vi "get_schemas.vi"(8 "error in (no error)":errorcluster, 11 "DB Session ID":i32) -> (0 "error out":errorcluster, 2 "Schemas":string[](array[string]), 3 "DB Session ID out":i32)   [LabVIEW 2017, in "Database.lvlib"]
uses:
  Database.lvlib
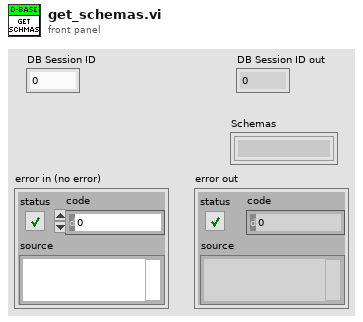
[diagram p1: front panel]
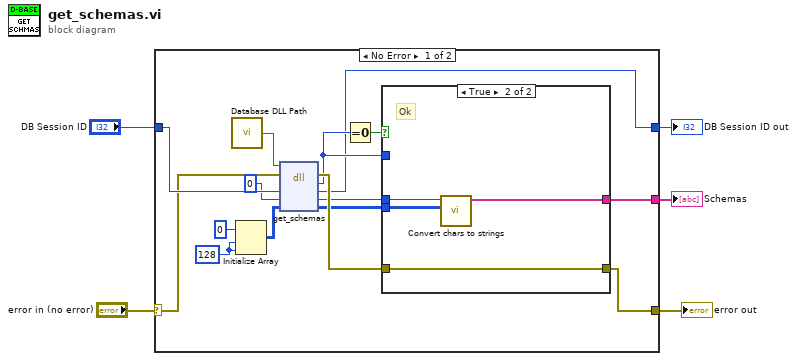
[diagram p0: block diagram]
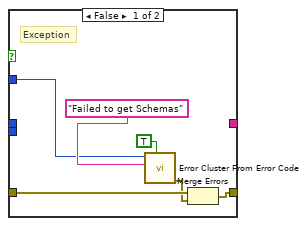
[diagram p2: hidden frame]
diagram:
  n1 = case shown="No Error" "error in (no error)" {
    selector: "error in (no error)" -> [w17 w32]
    tunnel: [w12 w32] -> w4
    tunnel: "DB Session ID" -> [w18 w31]
    tunnel: [w8 _] -> w2
    tunnel: [w6 w31] -> w1
    frame No Error {
      w14 = 128 ("dimension size")
      n2 = call "Database DLL Path.vi"() -> ("DLL Path"=w19:path)  [unwired: 5 in]
      n3 = Initialize Array(i8 0 ("element"), w14, w14) -> (w13:i8[][])
      n4 = dll-call lib="?" fn="get_schemas"(path in=w19, error in=w17, "session_id"=w18, "n_schemas"=0, "schemas"=w13) -> (error out=w20:errorcluster, "return type"=w7:i32, "session_id"=w6:i32, "n_schemas"=w11:i32, "schemas"=w9:i8[][])  [unwired: 1 in, 1 out]
      n5 = Equal To 0?(x=w7) -> (x = 0?=w10:bool)
      n6 = case shown="True" w10 {
        tunnel: w20 -> [w26 w30]
        tunnel: [w25 w30] -> w12
        tunnel: w11 -> [_ w29]
        tunnel: w9 -> [_ w28]
        tunnel: [_ w27] -> w8
        tunnel: w7 -> [w21 _]
        frame False {
          # "Exception"
          n7 = call <vilib>:"Error Cluster From Error Code.vi"("show call chain? (False)"=TRUE, "error message (\"\")"="Failed to get Schemas" ("error message (\"\")"), "error code (0)"=w21) -> ("error out"=w24:errorcluster)  [unwired: 6 in]
          n8 = Merge Errors(w26, w24) -> (w25:errorcluster)
        }
        frame True {
          # "Ok"
          n9 = call "Convert chars to strings.vi"("Char Array"=w28, "Array Length"=w29) -> ("Strings"=w27:string[])  [unwired: 9 in]
        }
      }
    }
    frame Error {
    }
  }
  "error out" <- w4
  "Schemas" <- w2
  "DB Session ID out" <- w1
